vi "Get Channel Data in By Channel ID.vi"(8 "error in (no error)":errorcluster, 9 "Channel IDs":T1[](array[typedef]) format="%.0x") -> (0 "error out":errorcluster, 1 "default values":dbl[](array[numeric]), 2 "FIFO indexes":i32[](array[numeric]), 4 "channel names":string[](array[string]))   [LabVIEW 2017, in "Routing and Faulting System Explorer.lvlib"]
uses:
  Routing and Faulting System Explorer.lvlib
  <vilib>/NI Veristand/Custom Device API/Custom Device Item Ref.ctl
  <vilib>/NI VeriStand/Custom Device API/Custom Device API.lvlib
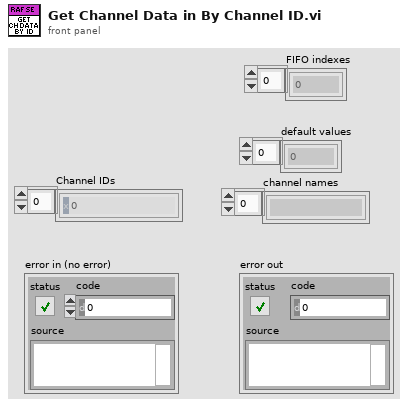
[diagram p1: front panel]
types:
  T1 = typedef "Custom Device API.lvlib/Custom Device Item Ref.ctl" = u64
  T2 = typedef "Custom Device API.lvlib/Custom Device Channel.ctl" = cluster{"Type":T3, "Units":string, "Default Value":dbl, "Faultable":bool, "Scalable":bool}
  T3 = typedef "Custom Device API.lvlib/Custom Device Channel Type.ctl" = enum16{"Input", "Output"}
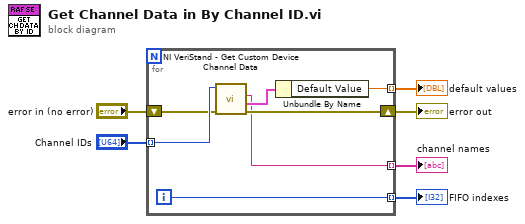
[diagram p0: block diagram]
diagram:
  n1 = for {
    shift-right: [w13] -> w5
    shift-left: "error in (no error)" -> [w7]
    tunnel: "Channel IDs" -> [w10] mode=indexing
    tunnel: [w11] -> w6 mode=indexing
    tunnel: [w9] -> w3 mode=indexing
    tunnel: [w8] -> w2 mode=indexing
    i -> [w8]
    n2 = call <vilib>:"NI VeriStand - Get Custom Device Channel Data.vi"("error in (no error)"=w7, "Channel Ref in"=w10) -> ("error out"=w13:errorcluster, "Channel"=w12:T2, "Channel Name"=w9:string)  [unwired: 4 in, 3 out]
    n3 = Unbundle By Name(w12) -> ("Default Value"=w11:dbl)
  }
  "default values" <- w6
  "error out" <- w5
  "FIFO indexes" <- w2
  "channel names" <- w3
